vi "Configure Audio Device.vi"(7 "Buffer Size (4096)":i32=4096, 8 "error in (no error)":errorcluster, 9 "Device Config":T1, 10 "Audio Device":T3={"Name"="", "ID"=[], "Device Type"=enum."Playback"}, 11 "Backend (Default)":T6=enum."Default") -> (0 "error out":errorcluster, 3 "Audio Device Refnum":T5)   [LabVIEW 2020, in "G-Audio.lvlib"]
doc: "Configure an audio device for playback or capture. If Backend is unwired, the default audio backend will be used. If Audio Device is unwired, the default device will be used for the specified backend.\n\nUse <b>Enumerate Audio Backend.vi</b> and <b>Enumerate Audio Device.vi</b> to query the available audio system."
uses:
  G-Audio.lvlib
  Controls/Backends.ctl
  Controls/Audio Device Refnum.ctl
  Controls/Audio Device Info.ctl
  Controls/Audio Device Type.ctl
  Controls/Audio Device Config.ctl
  Controls/Audio Device Format.ctl
  <vilib>/Utility/error.llb/Error Cluster From Error Code.vi
  lib/g_audio_x86.dll
  lib/g_audio_x64.dll
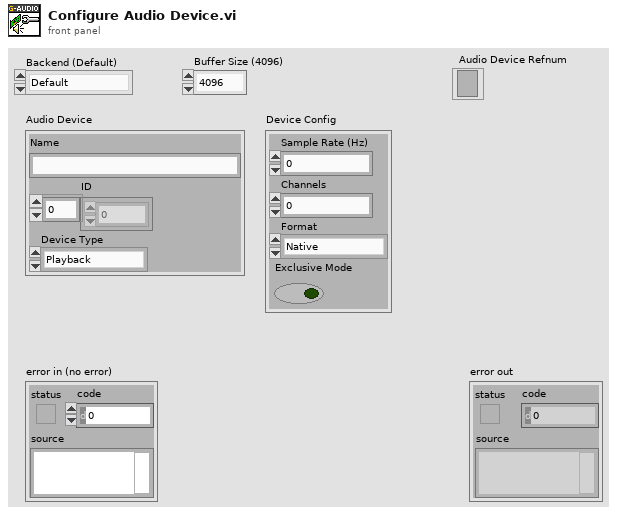
[diagram p1: front panel]
types:
  T1 = typedef "G-Audio.lvlib/Audio Device Config.ctl" = cluster{"Sample Rate (Hz)":u32, "Channels":u32, "Format":T2, "Exclusive Mode":bool}
  T2 = typedef "G-Audio.lvlib/Audio Device Format.ctl" = enum16{"Native", "U8", "I16", "I32", "SGL"}
  T3 = typedef "G-Audio.lvlib/Audio Device Info.ctl" = cluster{"Name":string, "ID":u8[], "Device Type":T4}
  T4 = typedef "G-Audio.lvlib/Audio Device Type.ctl" = enum16{"(None)", "Playback", "Capture", "Duplex", "Loopback"}
  T5 = typedef "G-Audio.lvlib/Audio Device Refnum.ctl" = refnum<file>
  T6 = typedef "G-Audio.lvlib/Backends.ctl" = enum16{"WASAPI", "DirectSound", "WinMM", "Core Audio", "sndio", "audio(4)", "OSS", "PulseAudio", "ALSA", "JACK", "AAudio", "OpenSL|ES", "Web Audio", "Custom", "Null", "Default"}
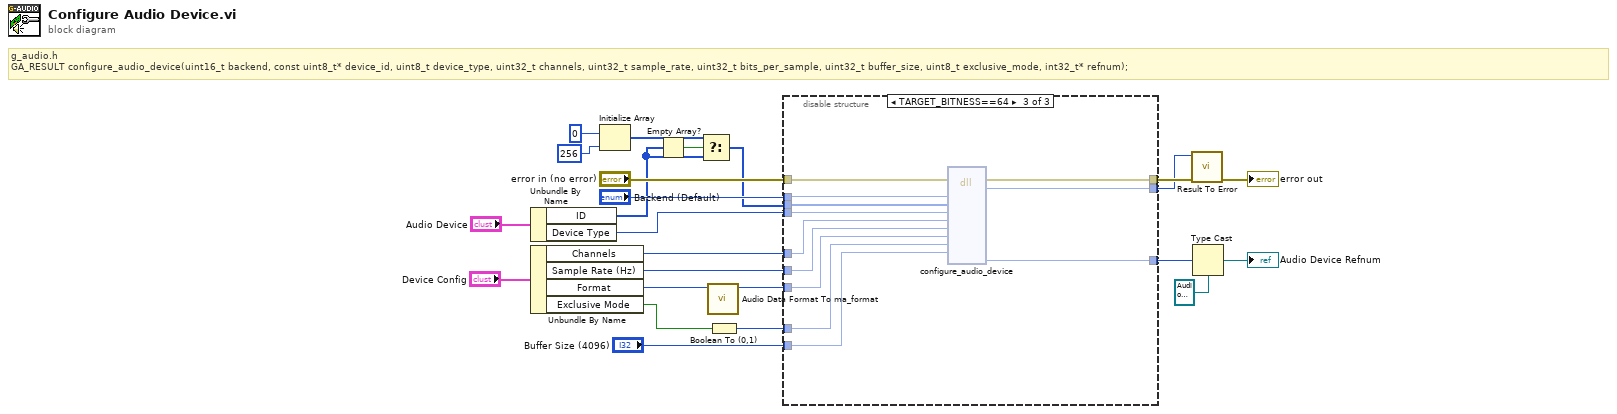
[diagram p0: block diagram]
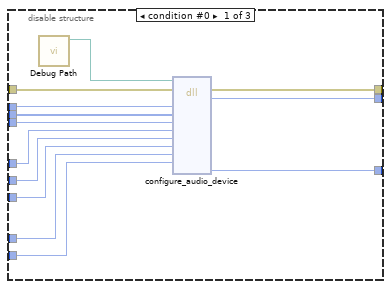
[diagram p2: hidden frame]
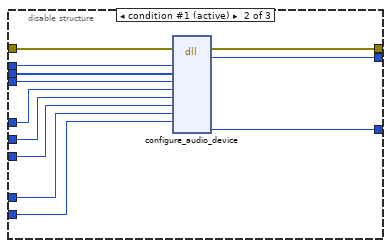
[diagram p3: hidden frame]
diagram:
  # "g_audio.h\nGA_RESULT configure_audio_device(uint16_t backend, const uint8_t* device_id, uint8_t device_type, uint32_t channels, uint32_t sample_rate, uint32_t bits_per_sample, uint32_t buffer_size, uint8_t exclusive_mode, int32_t* refnum);"
  n1 = Unbundle By Name("Audio Device") -> ("ID"=w3:u8[], "Device Type"=w14:T4)
  n2 = Unbundle By Name("Device Config") -> ("Channels"=w12:u32, "Sample Rate (Hz)"=w11:u32, "Format"=w10:T2, "Exclusive Mode"=w9:bool)
  n3 = Initialize Array(u8 0 ("dimension size"), 256 ("dimension size")) -> (w4:u8[])
  n4 = Empty Array?(array=w3) -> (empty?=w7:bool)
  n5 = Select(t=w4, s=w7, f=w3) -> (s? t:f=w2:u8[])
  n6 = call "Audio Data Format To ma_format.vi"("Format"=w10) -> ("ma_format"=w1:u16)  [unwired: 10 in]
  n7 = Boolean To (0,1)(Boolean=w9) -> (0, 1=w8:i16)
  n8 = disable-structure shown="TARGET_BITNESS==64" {
    disable-tunnel: "error in (no error)" -> [w33 w45 w57]
    disable-tunnel: [w37 w49 w61] -> w23
    disable-tunnel: "Backend (Default)" -> [w36 w48 w60]
    disable-tunnel: w2 -> [w32 w44 w56]
    disable-tunnel: [w35 w47 w59] -> w20
    disable-tunnel: [w34 w46 w58] -> w17
    disable-tunnel: "Buffer Size (4096)" -> [w31 w43 w55]
    disable-tunnel: w14 -> [w25 w38 w50]
    disable-tunnel: w12 -> [w30 w42 w54]
    disable-tunnel: w11 -> [w29 w41 w53]
    disable-tunnel: w1 -> [w28 w40 w52]
    disable-tunnel: w8 -> [w27 w39 w51]
    frame condition #0 {
      n9 = call "Debug Path.vi"() -> ("Debug Path"=w26:path)  [unwired: 11 in]
      n10 = dll-call lib="?" fn="configure_audio_device"(path in=w26, error in=w33, "backend_in"=w36, "device_id"=w32, "device_type"=w25, "channels"=w30, "sample_rate"=w29, "format"=w28, "exclusive_mode"=w27, "buffer_size"=w31) -> (error out=w37:errorcluster, "result"=w35:i32, "refnum"=w34:i32)  [unwired: 10 in, 1 out]
    }
    frame condition #1 (active) {
      n11 = dll-call lib="C:/github/dataflowg/g-audio/src/LabVIEW/G-Audio/lib/g_audio_x86.*" fn="configure_audio_device"(error in=w45, "backend_in"=w48, "device_id"=w44, "device_type"=w38, "channels"=w42, "sample_rate"=w41, "format"=w40, "exclusive_mode"=w39, "buffer_size"=w43) -> (error out=w49:errorcluster, "result"=w47:i32, "refnum"=w46:i32)  [unwired: 11 in, 1 out]
    }
    frame condition #2 {
      n12 = dll-call lib="C:/github/dataflowg/g-audio/src/LabVIEW/G-Audio/lib/g_audio_x64.*" fn="configure_audio_device"(error in=w57, "backend_in"=w60, "device_id"=w56, "device_type"=w50, "channels"=w54, "sample_rate"=w53, "format"=w52, "exclusive_mode"=w51, "buffer_size"=w55) -> (error out=w61:errorcluster, "result"=w59:i32, "refnum"=w58:i32)  [unwired: 11 in, 1 out]
    }
  }
  n13 = call "Result To Error.vi"("error in (no error)"=w23, "Result Code"=w20) -> ("error out"=→"error out":errorcluster)  [unwired: 9 in]
  n14 = Type Cast(type=T5 refnum ("Audio Device Refnum"), x=w17) -> (*(type *) &x=→"Audio Device Refnum":T5)
